vi "Get Top Level Path.vi"(8 "error in (no error)":errorcluster, 11 "Abstract Model in":refnum<class "Abstract Model.lvclass">) -> (0 "error out":errorcluster, 2 "Top Level Path":path, 3 "Abstract Model out":refnum<class "Abstract Model.lvclass">)   [LabVIEW 2013, in "Abstract Model.lvlib" / "Abstract Model.lvclass"]
uses:
  Abstract Model.lvclass
  Abstract Model.lvclass/Abstract Model.ctl
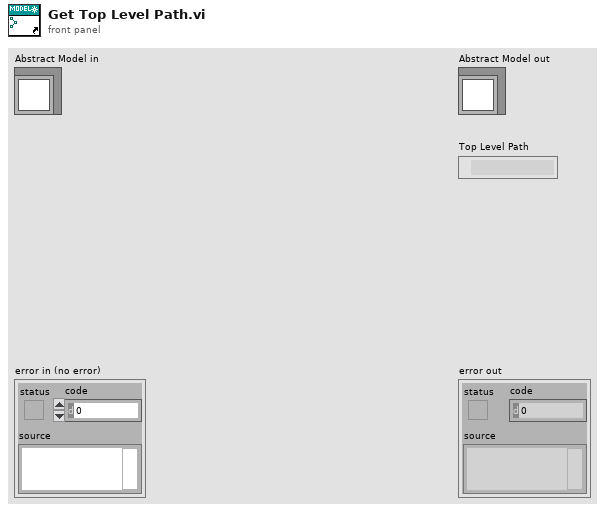
[diagram p1: front panel]
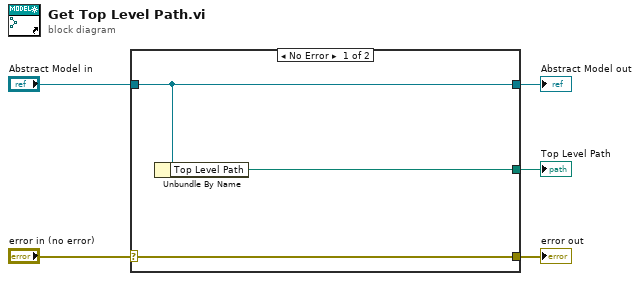
[diagram p0: block diagram]
diagram:
  n1 = case shown="No Error" "error in (no error)" {
    selector: "error in (no error)" -> [w8 w9]
    tunnel: [w8 w9] -> w4
    tunnel: [w7 w10] -> w2
    tunnel: "Abstract Model in" -> [w7 w10]
    tunnel: [w6 _] -> w1
    frame No Error {
      n2 = Unbundle By Name(w7) -> ("Top Level Path"=w6:path)
    }
    frame Error {
    }
  }
  "error out" <- w4
  "Abstract Model out" <- w2
  "Top Level Path" <- w1
